vi "Write Data Type.vi"(8 "error in (no error)":errorcluster, 10 "Data Type":T1, 11 "OnChange_Boolean in":refnum<class "OnChangeNotifier_DBL.lvclass">) -> (0 "error out":errorcluster, 3 "OnChange_Boolean out":refnum<class "OnChangeNotifier_DBL.lvclass">)   [LabVIEW 2021, in "OnChangeNotifier_DBL.lvclass"]
uses:
  OnChangeNotifier_DBL.lvclass
  Support/Class Type.ctl
  <vilib>/TSA/Abstract Data Classes/Abs_Types/Single Float/Abs_Single Float.lvclass
  OnChangeNotifier_DBL.lvclass/OnChangeNotifier_DBL.ctl
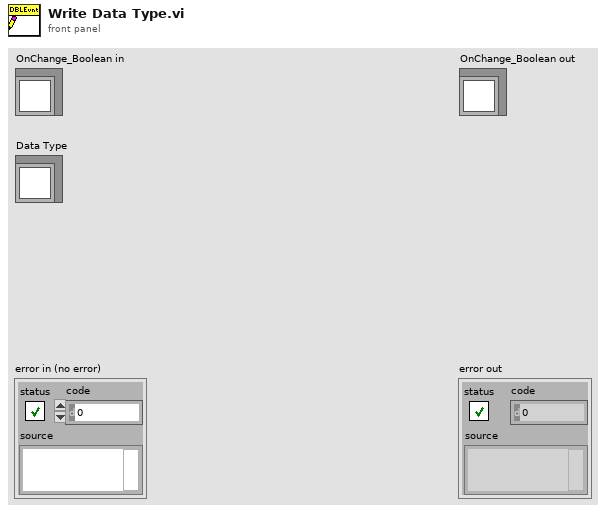
[diagram p1: front panel]
types:
  T1 = typedef "OnChangeNotifier_DBL.lvclass/Class Type.ctl" = refnum<class "Abs_Single Float.lvclass">
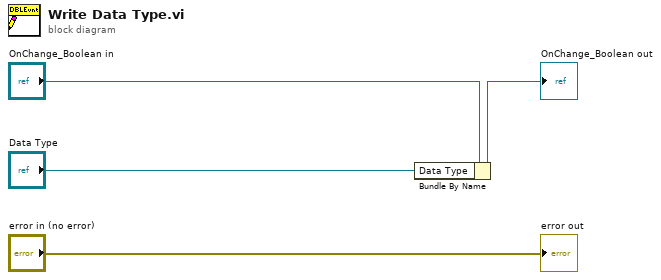
[diagram p0: block diagram]
diagram:
  n1 = Bundle By Name(cluster="OnChange_Boolean in", "Data Type"="Data Type") -> (→"OnChange_Boolean out":refnum<class "OnChangeNotifier_DBL.lvclass">)
  "error out" <- "error in (no error)"
